vi "DeleteDB.vi"() -> ()   [LabVIEW 2018]
uses:
  <vilib>/addons/database/Connection.llb/DB Tools Open Connec (Path).vi
  <vilib>/addons/database/NI_Database_API.lvlib
panel:
  in  "CheckNo":string
  out "error out":errorcluster
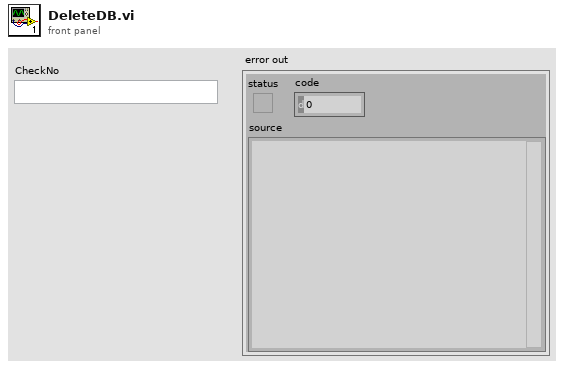
[diagram p1: front panel]
types:
  T1 = typedef "NI_Database_API.lvlib/Conn ObjectReference.ctl" = refnum<k1>
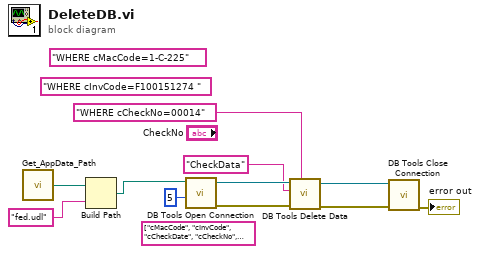
[diagram p0: block diagram]
diagram:
  (unwired) "WHERE cMacCode=1-C-225" ("condition")
  (unwired) "WHERE cInvCode=F100151274 " ("condition")
  (unwired) string[] ["cMacCode", "cInvCode", "cCheckDate", "cCheckNo", "cState", "cDefine1", "cDefine2", "cDefine3", "cDefine4", "cDefine5", "cDefine6", "cDefine7", "cDefine8", "cDefine9", "cDefine10", "cDefine11", "cDefine12", "cDefine13", "cDefine14", "cDefine15", "cDefine16", "cDefine17", "cDefine18"] ("Columns")
  n1 = call "Get_AppData_Path.vi"() -> ("path"=w10:path)  [unwired: 1 in]
  n2 = Build Path(base path=w10, name or relative path="fed.udl" ("名称或相对路径")) -> (appended path=w9:path)
  n3 = call-poly <vilib>:"DB Tools Open Connection.vi"("connection timeout (15)"=5, "connection information"=w9) -> ("error out"=w5:errorcluster, "connection reference"=w6:T1)  [unwired: 6 in]
  n4 = call <vilib>:"DB Tools Delete Data.vi"("condition"="WHERE cCheckNo=00014", "error in (no error)"=w5, "table"="CheckData", "connection reference"=w6) -> ("error out"=w4:errorcluster, "connection reference out"=w3:T1)  [unwired: 6 in]
  n5 = call <vilib>:"DB Tools Close Connection.vi"("error in (no error)"=w4, "connection reference"=w3) -> ("error out"=→"error out":errorcluster)  [unwired: 5 in]
